vi "single pullback.vi"() -> ()   [LabVIEW 2016]
uses:
  C:/Laser generated ultrasound/Labview/Kinesis Control/Thorlabs.MotionControl.KCube.BrushlessMotorCLI.dll
  Thorlabs.MotionControl.KCube.BrushlessMotorCLI.dll
  <vilib>/Utility/file.llb/Write To Spreadsheet File (DBL).vi
  <instrlib>/niScope/Acquire/Fetch/niScope Fetch.vi
  <instrlib>/niScope/Acquire/Fetch/niScope Multi Fetch.vi
  C:/Laser generated ultrasound/Labview/Kinesis Control/Thorlabs.MotionControl.Controls.dll
  Thorlabs.MotionControl.Controls.dll
panel:
  in  "Tab Control":T1(tab)
  in  "File Location":string="C:\\Laser generated ultrasound\\Labview\\Kinesis Control\\test data"
  in  "File name":string="scan_1"
  in  "SerialNumber":string="28251512"
  in  "Scan Length (mm)":dbl=20.0
  out "GetPositionCounter":sgl
  in  "Pullback speed (mm/s)":dbl=40.0
  in  "Repetition rate (Hz)":dbl=100.0
  in  "vertical range (V)":dbl=0.5 min=0.0 max=10.0 step=0.5
  in  "Depth (mm)":i32=15
  in  "Start acquisition":bool
  out "Number of samples":dbl
  out "number of a-lines":dbl
  out "?":cluster{dbl[], dbl[]}(graph)
  in  "Preview A-line?":bool
  in  "KCubeBrushlessControl":refnum<k24>(container)
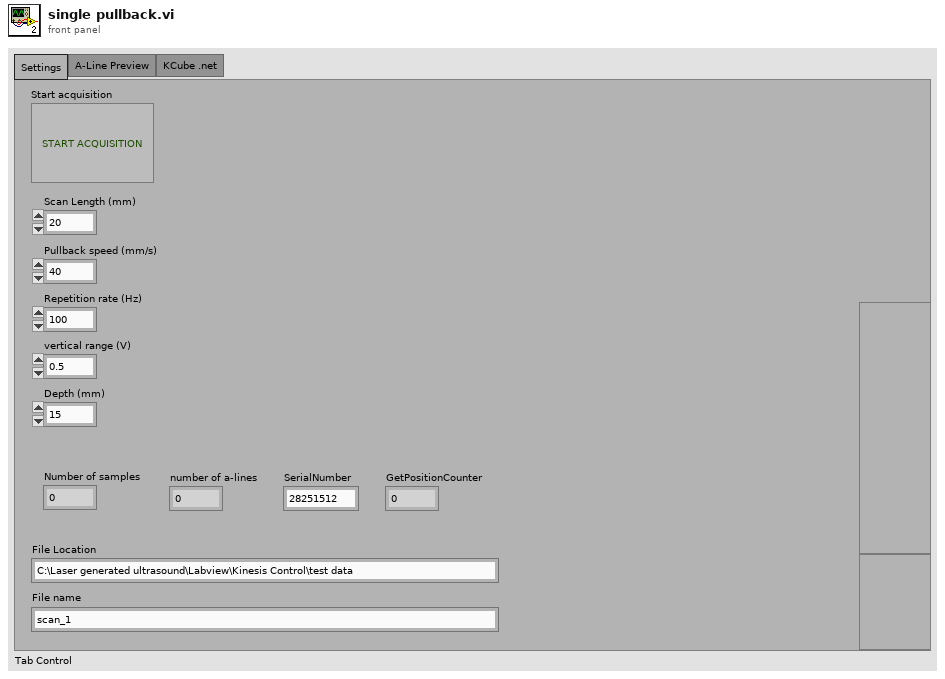
[diagram p1: front panel]
types:
  T1 = enum32{"Settings", "A-Line Preview", "KCube .net"}
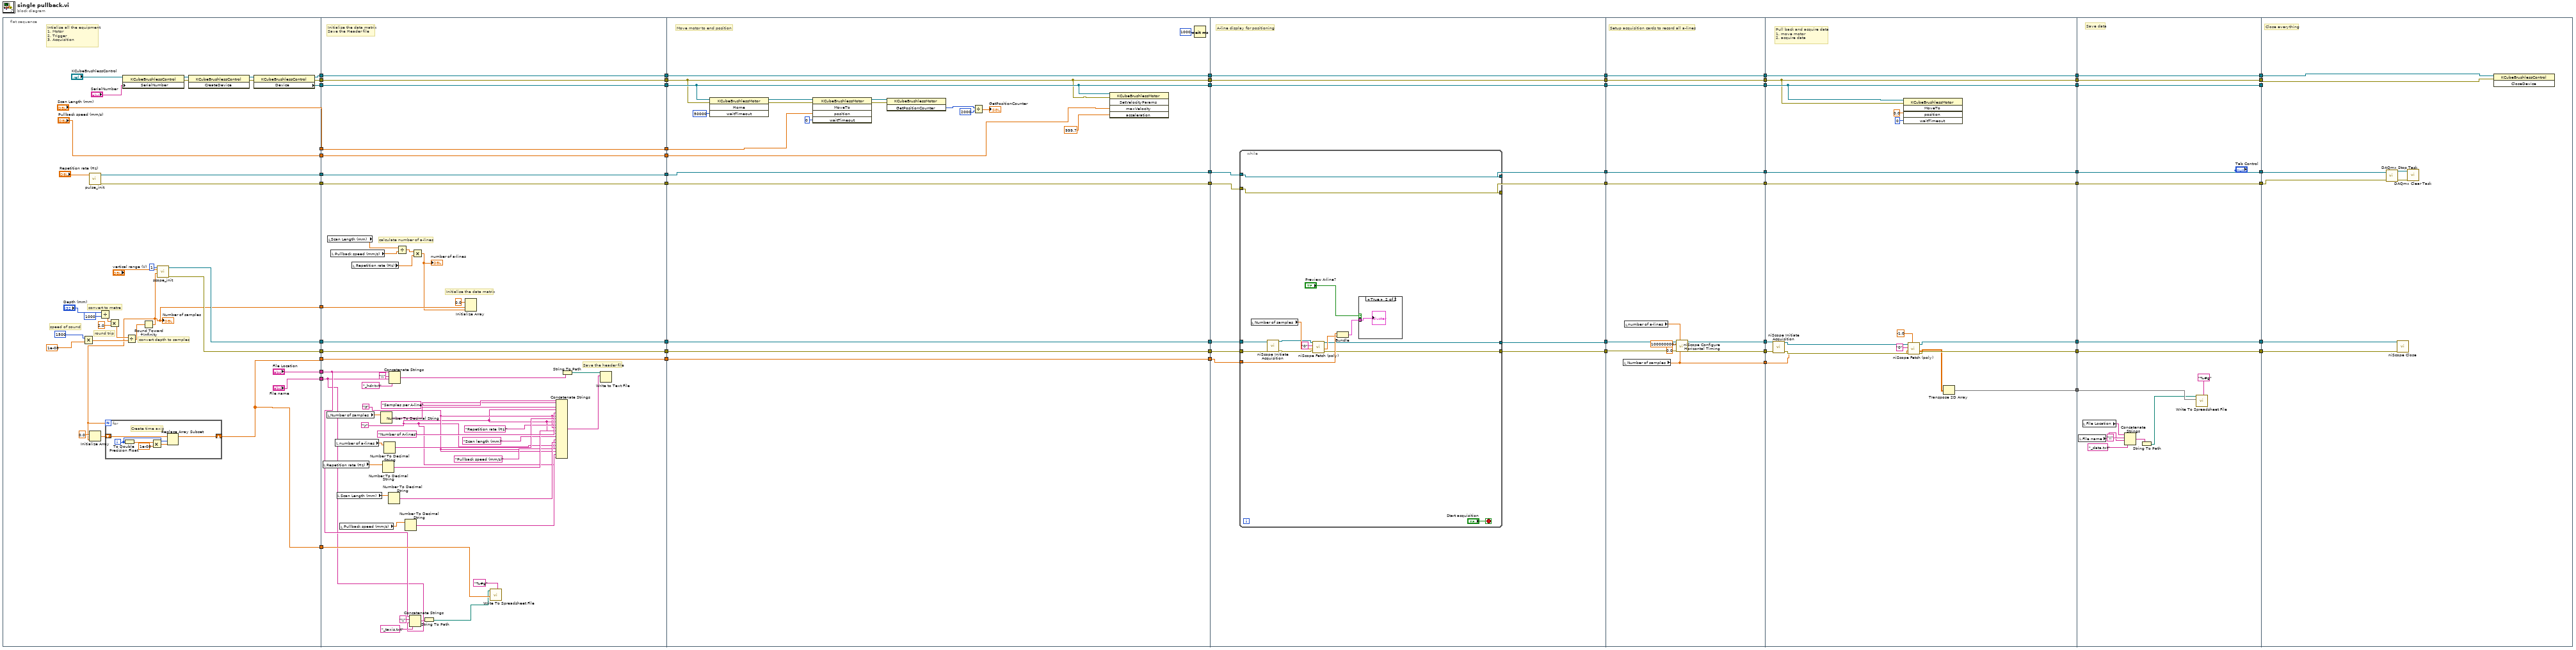
[diagram p0: block diagram]
diagram:
  n1 = flat-sequence {
    tunnel: [w89] -> w62
    tunnel: [w88] -> w60
    tunnel: [w87] -> w58
    tunnel: [w85] -> w56
    tunnel: [w84] -> w54
    tunnel: [w71] -> w52
    tunnel: [w72] -> w50
    tunnel: ["Scan Length (mm)"] -> w48
    tunnel: ["Pullback speed (mm/s)"] -> w46
    tunnel: [w63] -> w44
    tunnel: ["File Location"] -> w43
    tunnel: ["File name"] -> w42
    tunnel: [w64] -> w34
    tunnel: [w64] -> w31
    tunnel: w62 -> [w148]
    tunnel: [w148] -> w61
    tunnel: w60 -> [w147]
    tunnel: [w147] -> w59
    tunnel: w58 -> [w146]
    tunnel: [w146] -> w57
    tunnel: w56 -> [w145]
    tunnel: [w145] -> w55
    tunnel: w54 -> [w144]
    tunnel: [w144] -> w53
    tunnel: w52 -> [w143]
    tunnel: [w143] -> w51
    tunnel: w50 -> [w142]
    tunnel: [w142] -> w49
    tunnel: w48 -> [w141]
    tunnel: [w141] -> w47
    tunnel: w46 -> [w140]
    tunnel: [w140] -> w45
    tunnel: w44 -> [w138]
    tunnel: w43 -> [w103]
    tunnel: w42 -> [w102]
    tunnel: w34 -> [w110]
    tunnel: [w110] -> w33
    tunnel: w31 -> [w108]
    tunnel: w61 -> [w169]
    tunnel: w59 -> [w156]
    tunnel: w57 -> [w157]
    tunnel: [w169] -> w41
    tunnel: [w156] -> w40
    tunnel: [w157] -> w39
    tunnel: w55 -> [w155]
    tunnel: w53 -> [w154]
    tunnel: [w155] -> w38
    tunnel: [w154] -> w37
    tunnel: [w153] -> w36
    tunnel: w51 -> [w152]
    tunnel: [w152] -> w35
    tunnel: w49 -> [w153]
    tunnel: w47 -> [w151]
    tunnel: w45 -> [w150]
    tunnel: w33 -> [w149]
    tunnel: [w149] -> w32
    tunnel: w41 -> [w181]
    tunnel: [w181] -> w30
    tunnel: w40 -> [w180]
    tunnel: [w180] -> w28
    tunnel: w39 -> [w179]
    tunnel: [w179] -> w26
    tunnel: w38 -> [w178]
    tunnel: [w177] -> w24
    tunnel: w37 -> [w176]
    tunnel: [w175] -> w22
    tunnel: w36 -> [w174]
    tunnel: [w171] -> w20
    tunnel: w35 -> [w173]
    tunnel: [w170] -> w18
    tunnel: w32 -> [w172]
    tunnel: w30 -> [w210]
    tunnel: [w210] -> w29
    tunnel: w28 -> [w209]
    tunnel: [w209] -> w27
    tunnel: w26 -> [w208]
    tunnel: [w208] -> w25
    tunnel: w24 -> [w207]
    tunnel: [w207] -> w23
    tunnel: w22 -> [w206]
    tunnel: [w206] -> w21
    tunnel: w20 -> [w205]
    tunnel: [w203] -> w19
    tunnel: w18 -> [w204]
    tunnel: [w202] -> w17
    tunnel: [w198] -> w16
    tunnel: w29 -> [w228]
    tunnel: w27 -> [w224]
    tunnel: w25 -> [w225]
    tunnel: [w228] -> w15
    tunnel: [w224] -> w13
    tunnel: [w225] -> w11
    tunnel: w23 -> [w223]
    tunnel: w21 -> [w222]
    tunnel: [w223] -> w9
    tunnel: [w222] -> w7
    tunnel: [w214] -> w5
    tunnel: [w213] -> w3
    tunnel: w19 -> [w221]
    tunnel: w17 -> [w220]
    tunnel: w16 -> [w215]
    tunnel: [w211] -> w1
    tunnel: w15 -> [w243]
    tunnel: [w243] -> w14
    tunnel: w13 -> [w242]
    tunnel: [w242] -> w12
    tunnel: w11 -> [w241]
    tunnel: [w241] -> w10
    tunnel: w9 -> [w240]
    tunnel: [w240] -> w8
    tunnel: w7 -> [w239]
    tunnel: [w239] -> w6
    tunnel: w5 -> [w238]
    tunnel: [w238] -> w4
    tunnel: w3 -> [w237]
    tunnel: [w237] -> w2
    tunnel: w1 -> [w235]
    tunnel: w14 -> [w245]
    tunnel: w12 -> [w244]
    tunnel: w10 -> [_]
    tunnel: w8 -> [w249]
    tunnel: w6 -> [w248]
    tunnel: w4 -> [w247]
    tunnel: w2 -> [w246]
    frame #0 {
      # "round trip"
      # "speed of sound"
      # "convert depth to samples"
      # "convert to metre"
      # "Intialise all the equipment\n1. Motor\n2. Trigger\n3. Acquisition"
      n2 = Multiply(x=1500 ("y"), y=1e-08) -> (x*y=w76:dbl)
      n3 = call "pulse_init.vi"("Repetition rate"="Repetition rate (Hz)") -> ("error out"=w84:errorcluster, "Refnum out"=w85:refnum<k21>)  [unwired: 9 in]
      n4 = Divide(x="Depth (mm)", y=1000) -> (x/y=w75:dbl)
      n5 = Multiply(x=w75, y=2.0) -> (x*y=w73:dbl)
      n6 = property class="KCubeBrushlessControl"(reference="KCubeBrushlessControl", "SerialNumber"="SerialNumber") -> (reference out=w93:refnum<k24>, error out=w92:errorcluster)  [unwired: 1 in]
      n7 = Divide(x=w73, y=w76) -> (x/y=w79:dbl)
      n8 = Round Toward +Infinity(x=w79) -> (ceil(x): smallest int >= x=w63:dbl)
      "Number of samples" <- w63
      n9 = Initialize Array(0.0 ("element"), w63) -> (w65:dbl[])
      n10 = for {
        N: w63 -> [_]
        shift-right: [w101] -> w64
        shift-left: w65 -> [w100]
        i -> [w99]
        # "Create time axis"
        n11 = To Double Precision Float(number=w99) -> (double precision float=w98:dbl)
        n12 = Multiply(x=w98, y=1e-08) -> (x*y=w96:dbl)
        n13 = Replace Array Subset(array=w100, new element=w96, index=w99) -> (w101:dbl[])
      }
      n14 = call "scope_init.vi"("Num Samples"=w63, "vertical range"="vertical range (V)", "Averages"=1) -> ("error out"=w71:errorcluster, "IVI Refnum out"=w72:refnum<k15>)  [unwired: 7 in]
      n15 = invoke class="KCubeBrushlessControl" method="CreateDevice"(reference=w93, error in=w92) -> (reference out=w91:refnum<k24>, error out=w90:errorcluster)  [unwired: 1 in, 1 out]
      n16 = property class="KCubeBrushlessControl"(reference=w91, error in=w90) -> (reference out=w89:refnum<k24>, error out=w88:errorcluster, "Device"=w87:refnum<k24>)
    }
    frame #1 {
      w111 = "\r"
      w114 = "\t"
      # "Save the header file"
      # "Initialise the data matrix"
      # "calculate number of a-lines"
      # "Initialise the data matrix\nSave the Header file"
      n17 = local read "Repetition rate (Hz)"() -> (w120:dbl)
      n18 = local read "Number of samples"() -> (w126:dbl)
      n19 = local read "Scan Length (mm)"() -> (w137:dbl)
      n20 = local read "Pullback speed (mm/s)"() -> (w136:dbl)
      n21 = local read "number of a-lines"() -> (w123:dbl)
      n22 = local read "Scan Length (mm)"() -> (w117:dbl)
      n23 = local read "Pullback speed (mm/s)"() -> (w113:dbl)
      n24 = local read "Repetition rate (Hz)"() -> (w134:dbl)
      n25 = Number To Decimal String(number=w126) -> (decimal integer string=w125:string)  [unwired: 1 in]
      n26 = Number To Decimal String(number=w120) -> (decimal integer string=w119:string)  [unwired: 1 in]
      n27 = Number To Decimal String(number=w123) -> (decimal integer string=w122:string)  [unwired: 1 in]
      n28 = Number To Decimal String(number=w117) -> (decimal integer string=w116:string)  [unwired: 1 in]
      n29 = Concatenate Strings(w103, "\\" ("string"), w102, "_hdr.txt" ("string")) -> (w131:string)
      n30 = Divide(x=w137, y=w136) -> (x/y=w135:dbl)
      n31 = Number To Decimal String(number=w113) -> (decimal integer string=w112:string)  [unwired: 1 in]
      n32 = Concatenate Strings(w103, "\\" ("string"), w102, "_taxis.txt" ("string")) -> (w107:string)
      n33 = Multiply(x=w135, y=w134) -> (x*y=w133:dbl)
      "number of a-lines" <- w133
      n34 = String To Path(string=w107) -> (path=w104:path)
      n35 = Initialize Array(0.0 ("element"), w138, w133) -> ()  [unwired: 1 out]
      n36 = call-poly <vilib>:"Write To Spreadsheet File.vi"("format (%.3f)"="%#g", "1D data"=w108, "file path (dialog if empty)"=w104) -> ()  [unwired: 5 in, 1 out]
      n37 = Concatenate Strings("Samples per A-line" ("string"), w114, w125, w111, "Number of A-lines" ("string"), w114, w122, w111, "Repetition rate (Hz)" ("string"), w114, w119, w111, "Scan length (mm)" ("string"), w114, w116, w111, "Pullback speed (mm/s)" ("string"), w114, w112, w111) -> (w128:string)
      n38 = String To Path(string=w131) -> (path=w132:path)
      n39 = Write to Text File(file (use dialog)=w132, text=w128) -> ()  [unwired: 2 in, 3 out]
    }
    frame #2 {
      # "Move motor to end position"
      n40 = invoke class="KCubeBrushlessMotor" method="Home"(reference=w157, error in=w156, "waitTimeout"=50000) -> (reference out=w167:refnum<k24>, error out=w166:errorcluster)  [unwired: 1 in, 2 out]
      n41 = invoke class="KCubeBrushlessMotor" method="MoveTo"(reference=w167, error in=w166, "position"=w151, "waitTimeout"=0) -> (reference out=w164:refnum<k24>, error out=w163:errorcluster)  [unwired: 1 in, 3 out]
      n42 = invoke class="KCubeBrushlessMotor" method="GetPositionCounter"(reference=w164, error in=w163) -> ("GetPositionCounter"=w160:i32)  [unwired: 1 in, 2 out]
      n43 = Divide(x=w160, y=2000) -> (x/y=→"GetPositionCounter":dbl)
      n44 = invoke class="KCubeBrushlessMotor" method="SetVelocityParams"(reference=w157, error in=w156, "maxVelocity"=w150, "acceleration"=999.7) -> ()  [unwired: 1 in, 5 out]
      n45 = Wait (ms)(milliseconds to wait=u32 1000) -> ()  [unwired: 1 out]
    }
    frame #3 {
      # "A-line display for positioning"
      n46 = while {
        tunnel: w178 -> [w196]
        tunnel: w176 -> [w195]
        tunnel: [w196] -> w177
        tunnel: [w195] -> w175
        tunnel: w174 -> [w192]
        tunnel: w173 -> [w191]
        tunnel: w172 -> [w186]
        tunnel: [w183] -> w171
        tunnel: [w182] -> w170
        stop <- "Start acquisition" stop-if-true
        n47 = local read "Number of samples"() -> (w194:dbl)
        n48 = call <instrlib>:"niScope Initiate Acquisition.vi"("instrument handle"=w192, "error in"=w191) -> ("instrument handle out"=w190:refnum<k15>, "error out"=w189:errorcluster)  [unwired: 12 in]
        n49 = call-poly <instrlib>:"niScope Fetch (poly).vi"("error in"=w189, "numSamples"=w194, "channels"="0", "instrument handle"=w190) -> ("error out"=w182:errorcluster, "wfm"=w188:dbl[], "instrument handle out"=w183:refnum<k15>)  [unwired: 4 in, 1 out]
        n50 = Bundle(w186, "wfm"=w188) -> (w187:cluster{dbl[], "wfm":dbl[]})  [unwired: 1 in]
        n51 = case shown="True" "Preview A-line?" {
          tunnel: w187 -> [_ w197]
          frame False {
          }
          frame True {
            "?" <- w197
          }
        }
      }
    }
    frame #4 {
      # "Setup acquisition cards to record all a-lines"
      n52 = local read "Number of samples"() -> (w198:dbl)
      n53 = local read "number of a-lines"() -> (w199:dbl)
      n54 = call <instrlib>:"niScope Configure Horizontal Timing.vi"("instrument handle"=w205, "number of records"=w199, "min sample rate"=100000000.0, "reference position"=0.0, "error in"=w204, "min record length"=w198) -> ("instrument handle out"=w203:refnum<k15>, "error out"=w202:errorcluster)  [unwired: 8 in]
    }
    frame #5 {
      # "Pull back and acquire data\n1. move motor\n2. acquire data"
      n55 = call <instrlib>:"niScope Initiate Acquisition.vi"("instrument handle"=w221, "error in"=w220) -> ("instrument handle out"=w219:refnum<k15>, "error out"=w218:errorcluster)  [unwired: 12 in]
      n56 = invoke class="KCubeBrushlessMotor" method="MoveTo"(reference=w225, error in=w224, "position"=0.0, "waitTimeout"=0) -> ()  [unwired: 1 in, 5 out]
      n57 = call-poly <instrlib>:"niScope Fetch (poly).vi"("timeout"=-1.0, "error in"=w218, "numSamples"=w215, "channels"="0", "instrument handle"=w219) -> ("error out"=w213:errorcluster, "wfm"=w212:dbl[][], "instrument handle out"=w214:refnum<k15>)  [unwired: 3 in, 1 out]
      n58 = Transpose 2D Array(2D array=w212) -> (transposed array=w211:dbl[][])
    }
    frame #6 {
      # "Save data"
      n59 = local read "File name"() -> (w229:string)
      n60 = local read "File Location"() -> (w230:string)
      n61 = Concatenate Strings(w230, "\\" ("string"), w229, "_data.txt" ("string")) -> (w234:string)
      n62 = String To Path(string=w234) -> (path=w231:path)
      n63 = call-poly <vilib>:"Write To Spreadsheet File.vi"("format (%.3f)"="%#g", "2D data"=w235, "file path (dialog if empty)"=w231) -> ()  [unwired: 5 in, 1 out]
    }
    frame #7 {
      # "Close everything"
      n64 = call <vilib>:"DAQmx Stop Task.vi"("task/channels in"=w249, "error in"=w248) -> ("task out"=w251:refnum<k21>, "error out"=w250:errorcluster)  [unwired: 12 in]
      n65 = call <instrlib>:"niScope Close.vi"("instrument handle"=w247, "error in"=w246) -> ()  [unwired: 13 in, 1 out]
      n66 = call <vilib>:"DAQmx Clear Task.vi"("task in"=w251, "error in"=w250) -> ()  [unwired: 13 in, 1 out]
      n67 = invoke class="KCubeBrushlessControl" method="CloseDevice"(reference=w245, error in=w244) -> ()  [unwired: 1 in, 3 out]
    }
  }
